vi "Core_Record.vi"(8 "error in (no error)":errorcluster, 10 "Notifier Data":T1={"Notifier Type"=enum."Receive Message", "Data"=variant, "Time"=timestamp(0 s since 1904-01-01)}, 11 "HSMS Class in":refnum<class "HSMS Class.lvclass">) -> (0 "error out":errorcluster, 3 "HSMS Class out":refnum<class "HSMS Class.lvclass">)   [LabVIEW 2020, in "SECS Communication.lvlib" / "HSMS Class.lvclass"]
uses:
  HSMS Class.lvclass
  Notifier Data.ctl
  Notifier Type.ctl
  HSMS Class.lvclass/HSMS Class.ctl
  Read Log Path.vi
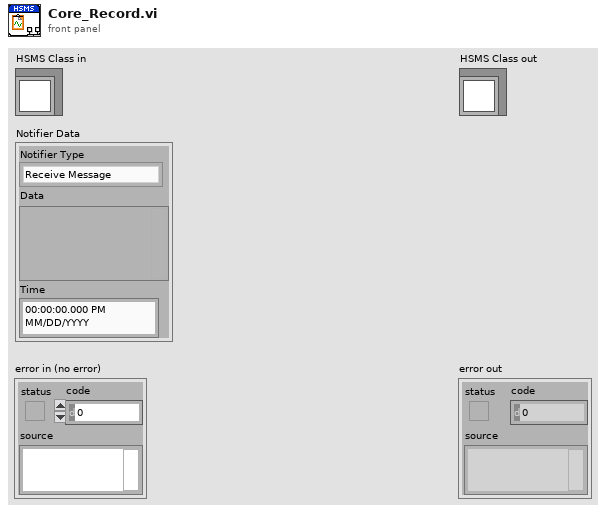
[diagram p1: front panel]
types:
  T1 = typedef "SECS Communication.lvlib/HSMS Class.lvclass/Notifier Data.ctl" = cluster{"Notifier Type":T2, "Data":variant, "Time":timestamp}
  T2 = typedef "SECS Communication.lvlib/HSMS Class.lvclass/Notifier Type.ctl" = enum16{"TCPIP Connect", "TCPIP Disconnect", "Receive Message", "Send Message", "T3 Timeout", "T6 Timeout", "T7 Timeout", "Error", "Stop"}
  T3 = enum16{"open", "replace", "create", "open or create", "replace or create", "replace or create with confirmation"}
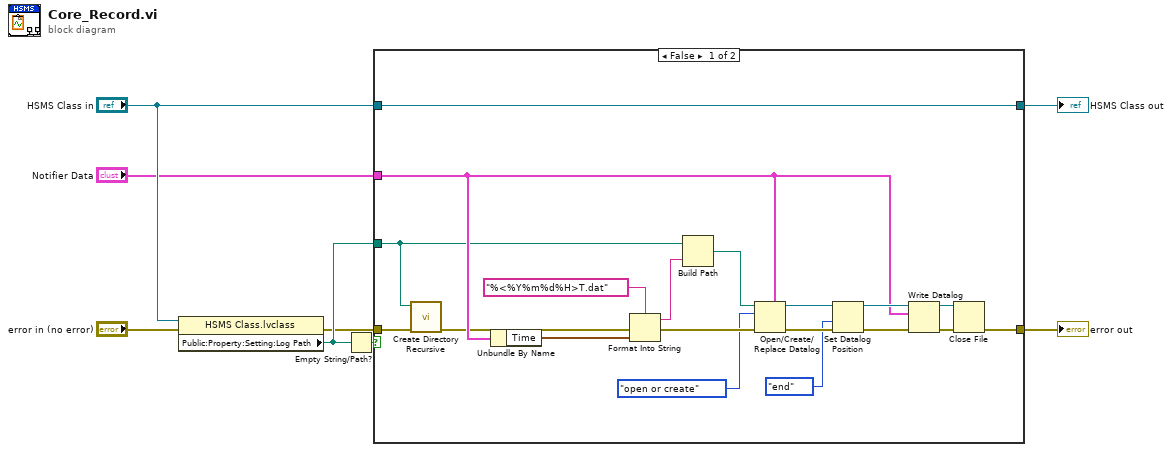
[diagram p0: block diagram]
diagram:
  n1 = property class="HSMS Class.lvclass"(reference="HSMS Class in", error in="error in (no error)") -> (error out=w6:errorcluster, "Public:Property:Setting:Log Path"=w8:path)  [unwired: 1 out]
  n2 = Empty String/Path?(string/path=w8) -> (empty?=w7:bool)
  n3 = case shown="False" w7 {
    tunnel: w8 -> [w10 _]
    tunnel: w6 -> [w11 w28]
    tunnel: "HSMS Class in" -> [w27 w29]
    tunnel: [w27 w29] -> w5
    tunnel: "Notifier Data" -> [w15 _]
    tunnel: [w12 w28] -> w4
    frame False {
      n4 = call <vilib>:"Create Directory Recursive.vi"("error in (no error)"=w11, "directory"=w10) -> ("error out"=w9:errorcluster)  [unwired: 3 in, 2 out]
      n5 = Unbundle By Name(w15) -> ("Time"=w26:timestamp)
      n6 = Format Into String(format string="%<%Y%m%d%H>T.dat", error in=w9, w26) -> (resulting string=w24:string, error out=w23:errorcluster)  [unwired: 1 in]
      n7 = Build Path(base path=w10, name or relative path=w24) -> (appended path=w22:path)
      n8 = Open/Create/Replace Datalog(5:w15, 8:w23, 10:T3."open or create" ("operation (0:open)"), 11:w22) -> (0:w19:errorcluster, 3:w20:refnum<k1>)  [unwired: 2 in, 1 out]
      n9 = Set Datalog Position(4:w19, 5:enum16{"start", "end", "current"}."end" ("from (0:start)"), 7:w20) -> (0:w16:errorcluster, 3:w17:refnum<k1>)  [unwired: 1 in]
      n10 = Write Datalog(4:w16, 6:w15, 7:w17) -> (0:w13:errorcluster, 3:w14:refnum<k1>)
      n11 = Close File(refnum=w14, error in=w13) -> (error out=w12:errorcluster)  [unwired: 1 out]
    }
    frame True {
    }
  }
  "error out" <- w4
  "HSMS Class out" <- w5
